vi "Concatenate Strings.vi"(8 "Numeric In":dbl, 10 "Description String":string="Higher Frequency:", 11 "Previous String":string="Higher Frequency:") -> (3 "Result String":string)   [LabVIEW 2014, in "ChirpEIS.lvclass"]
uses:
  ChirpEIS.lvclass
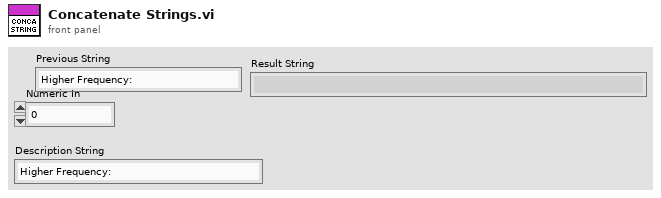
[diagram p1: front panel]
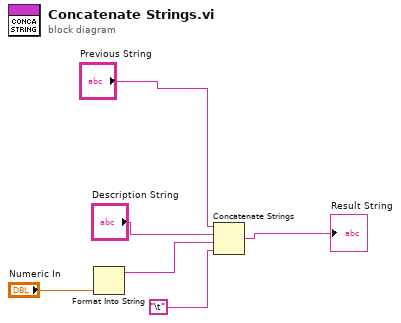
[diagram p0: block diagram]
diagram:
  n1 = Format Into String("Numeric In") -> (resulting string=w4:string)  [unwired: 3 in, 1 out]
  n2 = Concatenate Strings("Previous String", "Description String", w4, "\t") -> (→"Result String":string)
